vi "main.vi"() -> ()   [LabVIEW 2018]
doc: "This example demonstrates the use of binary morphological reconstruction in the particle analysis. The example allows you to keep the particles completely inside the ROI, completely outside the ROI or on the ROI."
uses:
  <vilib>/vision/NI_Vision_Development_Module.lvlib
panel:
  out "反射图":T1(plugin-control)
  in  "Font, Size & Style 3":T2={"Desired Font (Application)"=enum."Application Font", "[User-specified Font]"={"Font Name"="", "Size"=12, "Strikeout?"=FALSE, "Italic?"=FALSE, "Underline?"=FALSE, "Outline?"=FALSE, "Shadow?"=FALSE, "Bold?"=FALSE, "Rotation Angle"=0.0}, "Horizontal Alignment"=0, "Vertical Alignment"=0} {"Vertical Alignment" items=["Bottom", "Top", "Baseline"]; "Horizontal Alignment" items=["Left", "Center", "Right"]; "[User-specified Font]"."Rotation Angle" format="%.2f"}
  out "最大灰度值":sgl
  out "全图灰度级信息":T3 {"标准差" format="%.2f"; "均值" format="%.2f"; "相邻灰度级间隔" format="%.2f"; "起始灰度值" format="%.2f"; "最大值" format="%.2f"; "最小值" format="%.2f"}
  out "最大灰度值":sgl
  out "反射图灰度表":u32[](graph)
  in  "预处理":bool
  in  "查看标注":bool
  in  "导入图像":bool
  in  "删除标注":bool
  in  "退出":bool
  out "标注框总数":dbl
  out "全图灰度级信息":T3 {"标准差" format="%.2f"; "均值" format="%.2f"; "相邻灰度级间隔" format="%.2f"; "起始灰度值" format="%.2f"; "最大值" format="%.2f"; "最小值" format="%.2f"}
  out "穿透图灰度表":u32[](graph)
  in  "Font, Size & Style 2":T2={"Desired Font (Application)"=enum."Application Font", "[User-specified Font]"={"Font Name"="", "Size"=12, "Strikeout?"=FALSE, "Italic?"=FALSE, "Underline?"=FALSE, "Outline?"=FALSE, "Shadow?"=FALSE, "Bold?"=FALSE, "Rotation Angle"=0.0}, "Horizontal Alignment"=0, "Vertical Alignment"=0} {"Vertical Alignment" items=["Bottom", "Top", "Baseline"]; "Horizontal Alignment" items=["Left", "Center", "Right"]; "[User-specified Font]"."Rotation Angle" format="%.2f"}
  in  "Font, Size & Style":T2={"Desired Font (Application)"=enum."Application Font", "[User-specified Font]"={"Font Name"="", "Size"=12, "Strikeout?"=FALSE, "Italic?"=FALSE, "Underline?"=FALSE, "Outline?"=FALSE, "Shadow?"=FALSE, "Bold?"=FALSE, "Rotation Angle"=0.0}, "Horizontal Alignment"=0, "Vertical Alignment"=0} {"Vertical Alignment" items=["Bottom", "Top", "Baseline"]; "Horizontal Alignment" items=["Left", "Center", "Right"]; "[User-specified Font]"."Rotation Angle" format="%.2f"}
  out "框组":T4(array[cluster])
  in  "Operation":enum16{"overlay rectangle"}(ring)
  out "标注图":T1(plugin-control)
  # "穿透法图像"
  # "反射法图像"
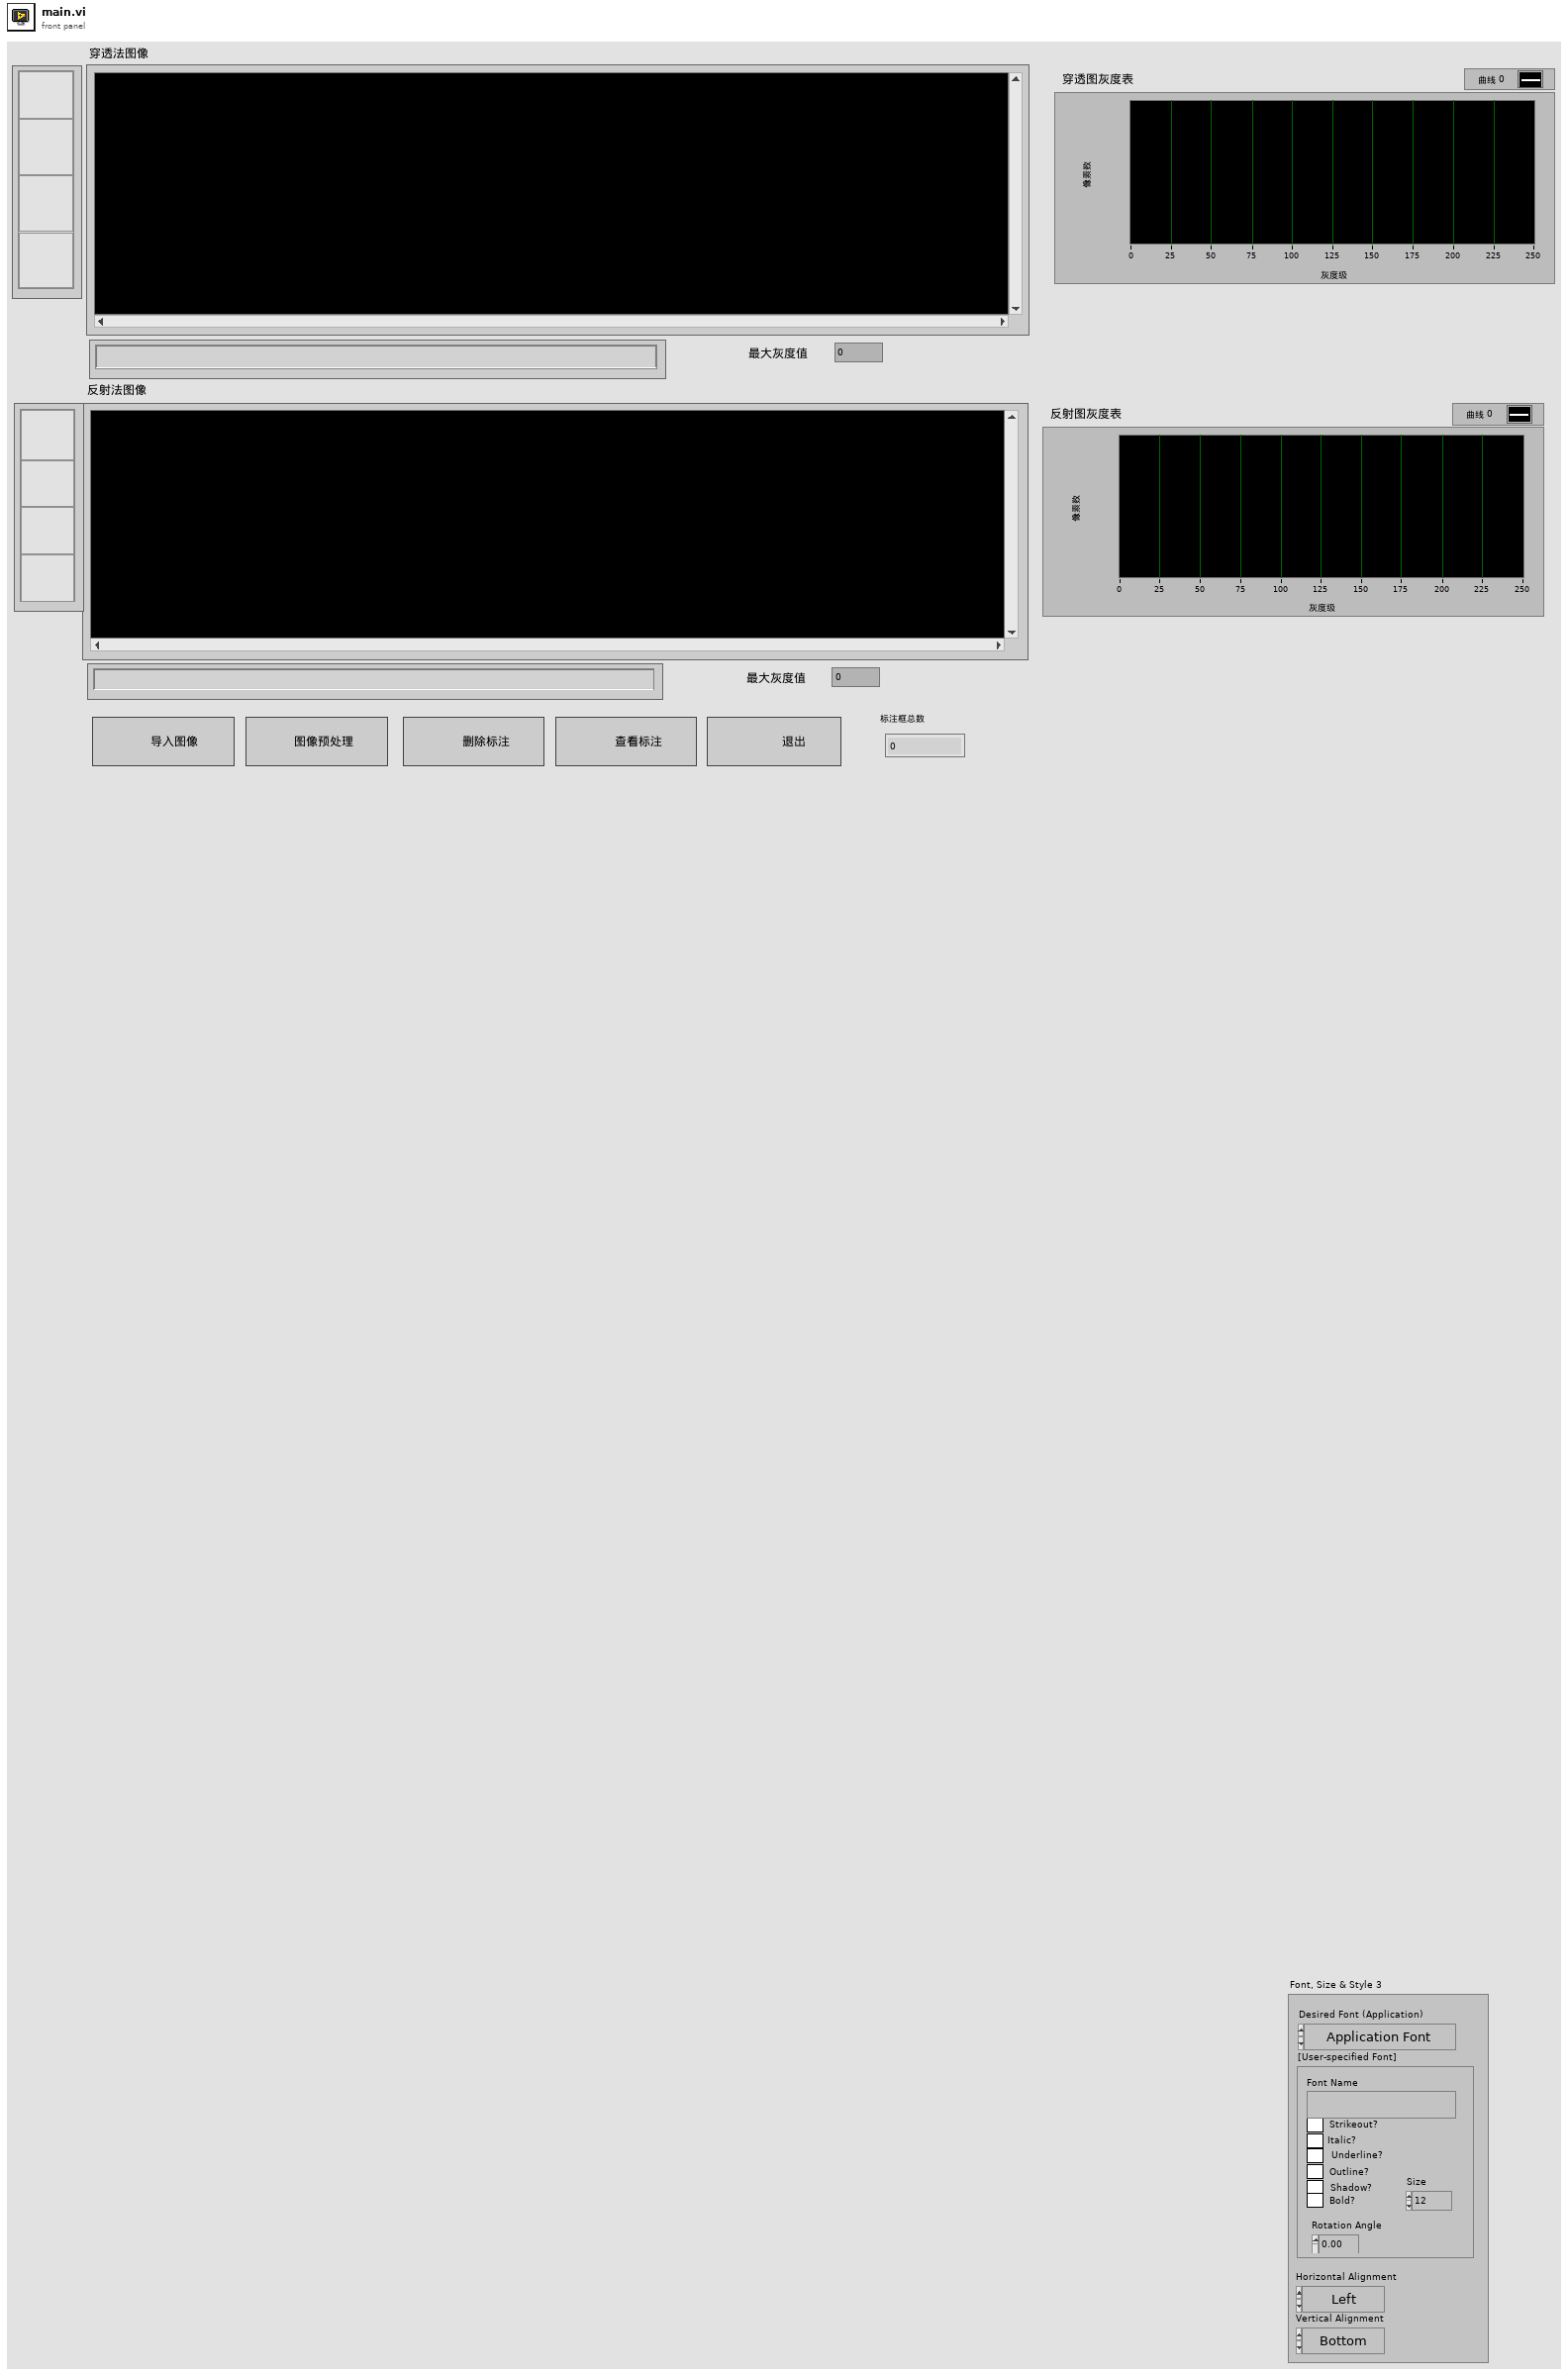
[diagram p1: front panel]
types:
  T1 = typedef "IMAQ Image.ctl" = refnum<image>
  T2 = cluster{"Desired Font (Application)":enum16{"User-specified Font", "Application Font", "System Font", "Dialog Font"}, "[User-specified Font]":cluster{"Font Name":string, "Size":i16, "Strikeout?":bool, "Italic?":bool, "Underline?":bool, "Outline?":bool, "Shadow?":bool, "Bold?":bool, "Rotation Angle":dbl}, "Horizontal Alignment":i16, "Vertical Alignment":i16}
  T3 = cluster{"histogram":u32[], "最小值":sgl, "最大值":sgl, "起始灰度值":sgl, "相邻灰度级间隔":sgl, "均值":sgl, "标准差":sgl, "像素面积":i32}
  T4 = cluster{"Global Rectangle":i32[], "Contours":cluster{"Contour Type":u32, "ROI Type":u32, "Points":i32[]}[]}[]
  T5 = typedef "Image Type" = u32
  T6 = cluster{"Global Rectangle":i32[], "Contours":cluster{"Contour Type":u32, "ROI Type":u32, "Points":i32[]}[]}
  T7 = cluster{"histogram":u32[], "Minimal Value":sgl, "Maximal Value":sgl, "Starting Value":sgl, "Interval Width":sgl, "Mean Value":sgl, "Standard  Variation":sgl, "Area (pixels)":i32}
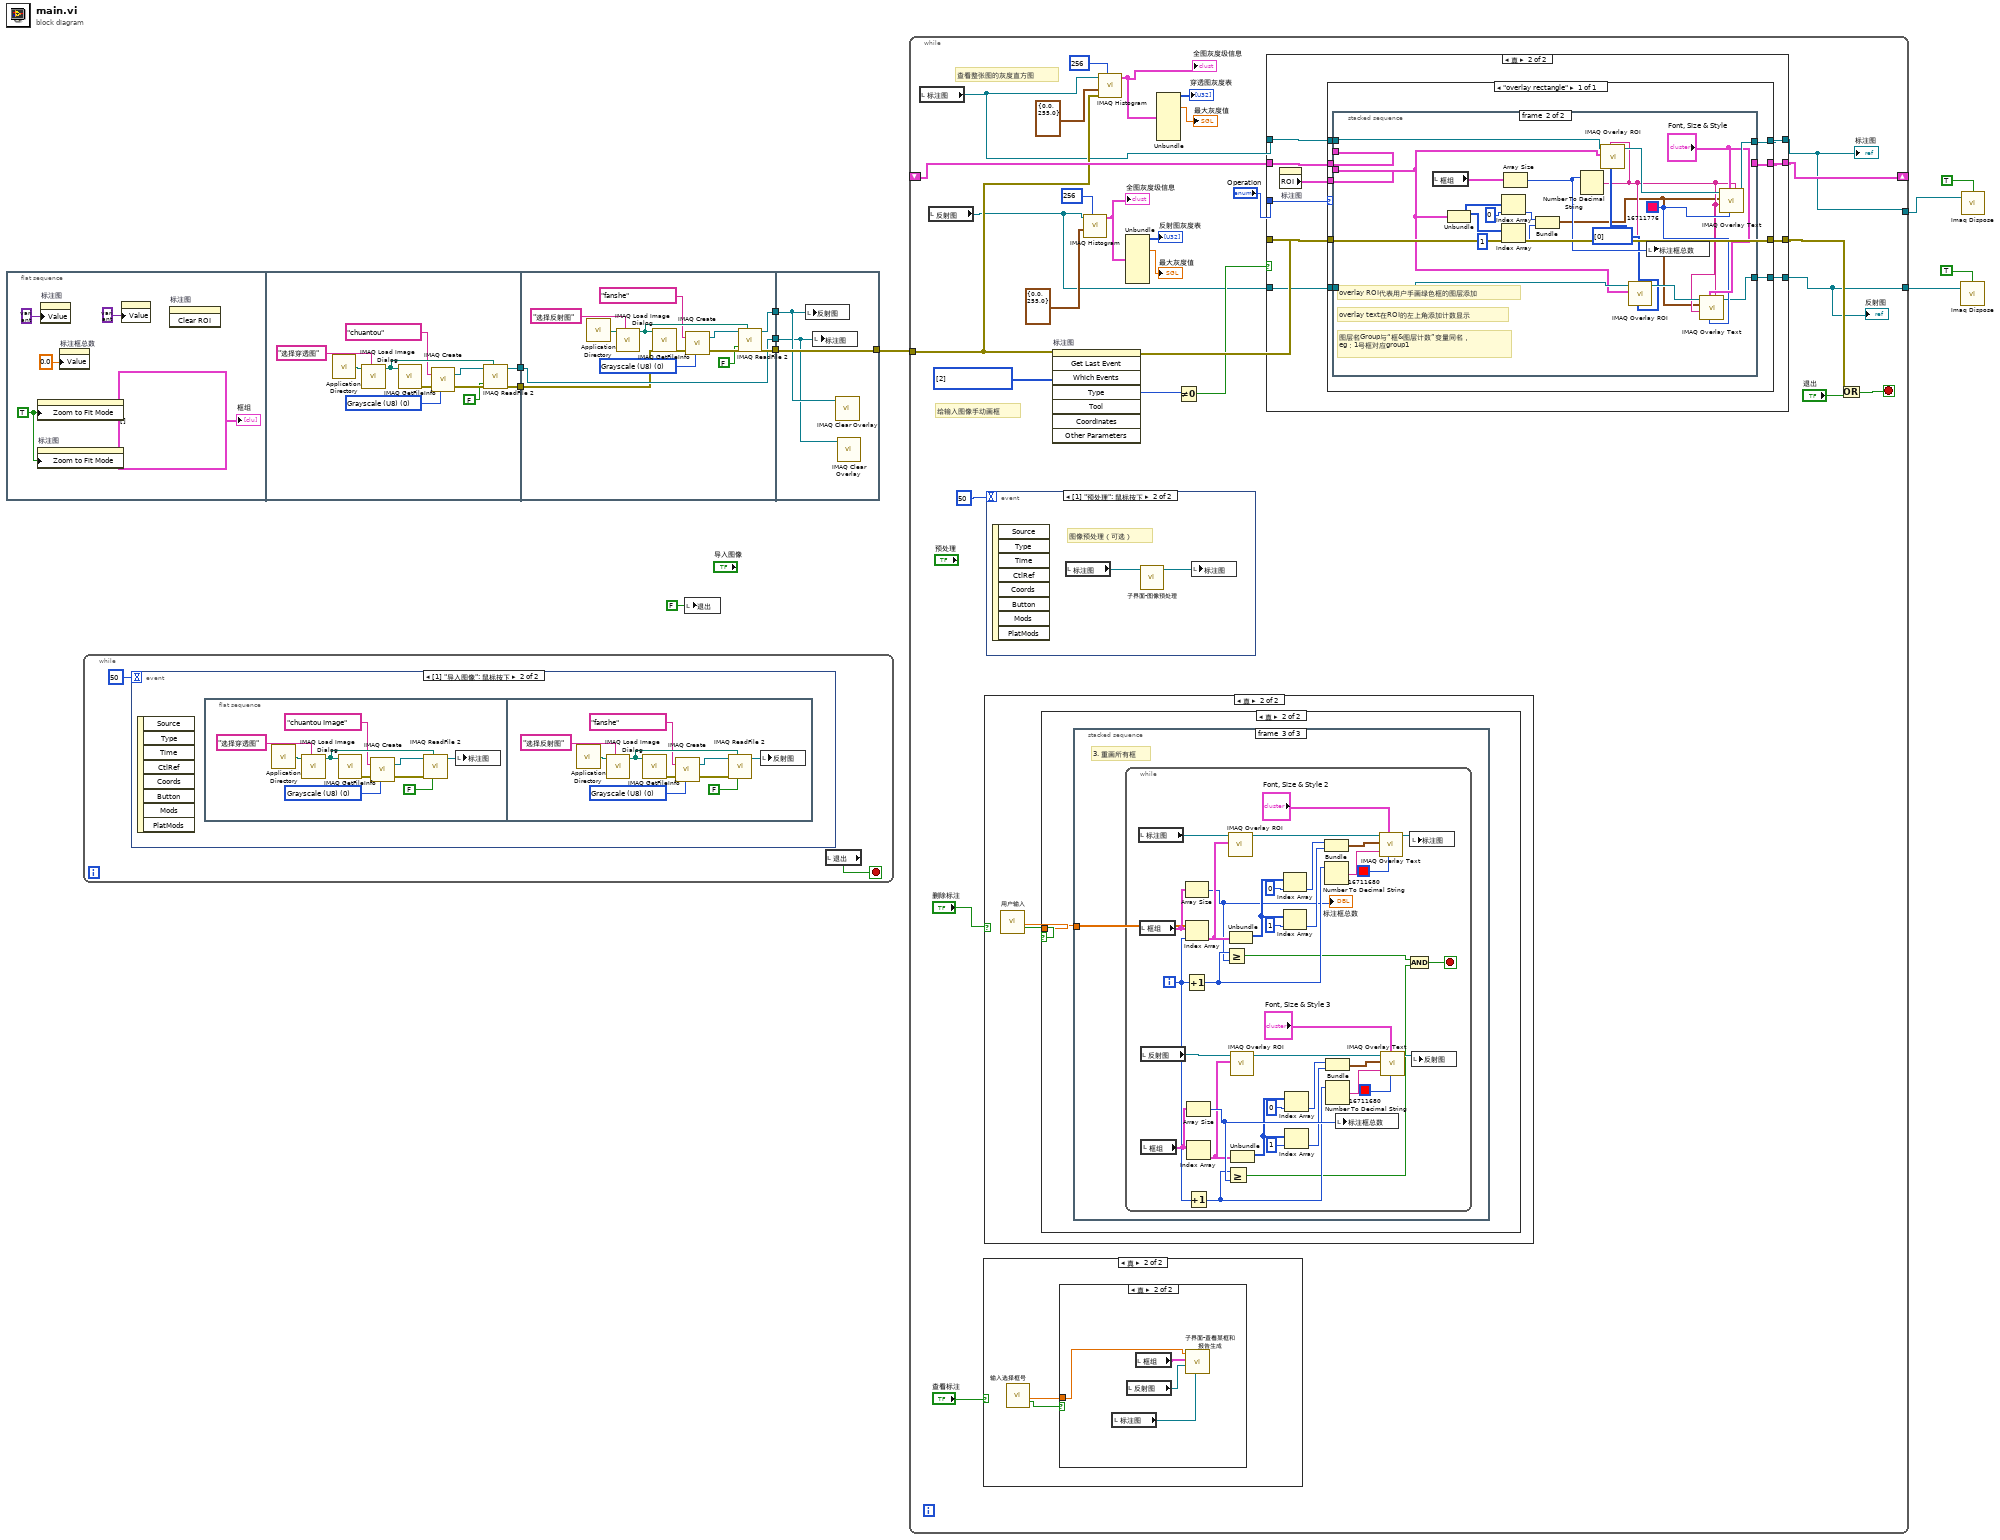
[diagram p0: block diagram]
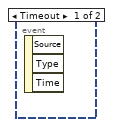
[diagram p2: hidden frame]
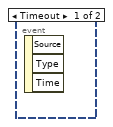
[diagram p3: hidden frame]
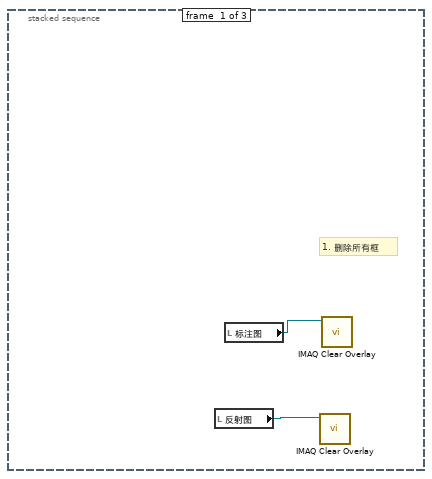
[diagram p8: hidden frame]
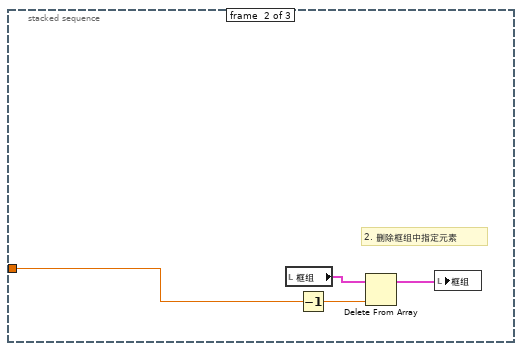
[diagram p9: hidden frame]
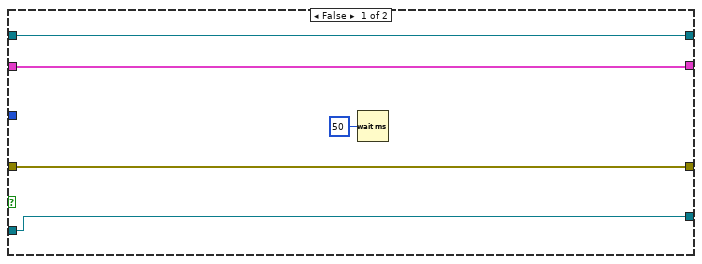
[diagram p10: hidden frame]
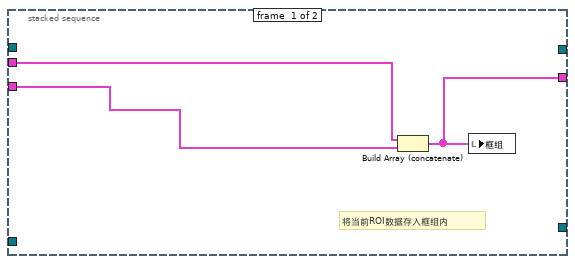
[diagram p11: hidden frame]
diagram:
  n1 = flat-sequence {
    tunnel: [w18] -> w8
    tunnel: [w17] -> w7
    tunnel: w8 -> [w29]
    tunnel: w7 -> [w30]
    tunnel: [w31] -> w6
    tunnel: [w30] -> w5
    tunnel: [w28] -> w4
    tunnel: [w43] -> w11
    tunnel: w6 -> [w43]
    tunnel: w5 -> [w41]
    tunnel: w4 -> [w42]
    frame #0 {
      w15 = TRUE ("Zoom to Fit Mode")
      n2 = property on="反射图" class="ImageControl"("Zoom to Fit Mode"=w15) -> ()  [unwired: 2 in, 2 out]
      n3 = property on="标注图" class="ImageControl"("Zoom to Fit Mode"=w15) -> ()  [unwired: 2 in, 2 out]
      n4 = property on="标注图" class="ImageControl"("Value"=variant ("值")) -> ()  [unwired: 2 in, 2 out]
      n5 = property on="标注框总数" class="DigNum (严格)"("Value"=0.0 ("标注框总数")) -> ()  [unwired: 2 in, 2 out]
      n6 = property on="反射图" class="ImageControl"("Value"=variant ("值")) -> ()  [unwired: 2 in, 2 out]
      n7 = invoke on="标注图" class="ImageControl" method="Clear ROI"() -> ()  [unwired: 3 in, 3 out]
      "框组" <- T4 [] ("框组")
    }
    frame #1 {
      w19 = T5 0 items=["Grayscale (U8)", "Grayscale (I16)", "Grayscale (SGL)", "Complex (CSG)", "RGB (U32)", "HSL (U32)", "RGB (U64)", "Grayscale (U16)"] ("Image Type")
      n8 = call <vilib>:"Application Directory.vi"() -> ("Application Directory"=w27:path)
      n9 = call "IMAQ Load Image Dialog"("Prompt"="选择穿透图" ("prompt"), "Start Path"=w27) -> ("Path"=w23:path)  [unwired: 7 in, 2 out]
      n10 = call "IMAQ GetFileInfo"("File Path"=w23) -> ("error out"=w24:errorcluster)  [unwired: 4 in, 6 out]
      n11 = call "IMAQ Create"("Image Name"="chuantou", "Image Type"=w19, "error in (no error)"=w24) -> ("New Image"=w25:T1, "error out"=w26:errorcluster)  [unwired: 2 in]
      n12 = call "IMAQ ReadFile 2"("Use File Path Image Type"=FALSE, "File Path"=w23, "error in (no error)"=w26, "Image"=w25) -> ("error out"=w18:errorcluster, "Image Out"=w17:T1)  [unwired: 3 in, 3 out]
    }
    frame #2 {
      w32 = T5 0 items=["Grayscale (U8)", "Grayscale (I16)", "Grayscale (SGL)", "Complex (CSG)", "RGB (U32)", "HSL (U32)", "RGB (U64)", "Grayscale (U16)"] ("Image Type")
      n13 = call <vilib>:"Application Directory.vi"() -> ("Application Directory"=w40:path)
      n14 = call "IMAQ Load Image Dialog"("Prompt"="选择反射图" ("prompt"), "Start Path"=w40) -> ("Path"=w36:path)  [unwired: 7 in, 2 out]
      n15 = call "IMAQ GetFileInfo"("error in (no error)"=w29, "File Path"=w36) -> ("error out"=w37:errorcluster)  [unwired: 3 in, 6 out]
      n16 = call "IMAQ Create"("Image Name"="fanshe", "Image Type"=w32, "error in (no error)"=w37) -> ("New Image"=w38:T1, "error out"=w39:errorcluster)  [unwired: 2 in]
      n17 = call "IMAQ ReadFile 2"("Use File Path Image Type"=FALSE, "File Path"=w36, "error in (no error)"=w39, "Image"=w38) -> ("error out"=w31:errorcluster, "Image Out"=w28:T1)  [unwired: 3 in, 3 out]
    }
    frame #3 {
      n18 = local write "反射图"(w42) -> ()
      n19 = local write "标注图"(w41) -> ()
      n20 = call "IMAQ Clear Overlay"("Image"=w42) -> ()  [unwired: 9 in, 2 out]
      n21 = call "IMAQ Clear Overlay"("Image"=w41) -> ()  [unwired: 9 in, 2 out]
    }
  }
  n22 = while {
    stop <- w44 stop-if-true
    n23 = event shown="[1] \"导入图像\": 鼠标按下" {
      selector: _ -> [_ _]
      dyn-events: _ -> [_ _]
      timeout: 50 -> [_ _]
      event Timeout {
        n24 = event-data() -> ()  [unwired: 1 in, 3 out]
      }
      event "导入图像": Mouse Down {
        n25 = event-data() -> ()  [unwired: 1 in, 8 out]
        n26 = flat-sequence {
          frame #0 {
            w47 = T5 0 items=["Grayscale (U8)", "Grayscale (I16)", "Grayscale (SGL)", "Complex (CSG)", "RGB (U32)", "HSL (U32)", "RGB (U64)", "Grayscale (U16)"] ("Image Type")
            n27 = call <vilib>:"Application Directory.vi"() -> ("Application Directory"=w55:path)
            n28 = call "IMAQ Load Image Dialog"("Prompt"="选择穿透图" ("prompt"), "Start Path"=w55) -> ("Path"=w51:path)  [unwired: 7 in, 2 out]
            n29 = call "IMAQ GetFileInfo"("File Path"=w51) -> ("error out"=w52:errorcluster)  [unwired: 4 in, 6 out]
            n30 = call "IMAQ Create"("Image Name"="chuantou Image", "Image Type"=w47, "error in (no error)"=w52) -> ("New Image"=w53:T1, "error out"=w54:errorcluster)  [unwired: 2 in]
            n31 = call "IMAQ ReadFile 2"("Use File Path Image Type"=FALSE, "File Path"=w51, "error in (no error)"=w54, "Image"=w53) -> ("Image Out"=w46:T1)  [unwired: 3 in, 4 out]
            n32 = local write "标注图"(w46) -> ()
          }
          frame #1 {
            w59 = T5 0 items=["Grayscale (U8)", "Grayscale (I16)", "Grayscale (SGL)", "Complex (CSG)", "RGB (U32)", "HSL (U32)", "RGB (U64)", "Grayscale (U16)"] ("Image Type")
            n33 = call <vilib>:"Application Directory.vi"() -> ("Application Directory"=w61:path)
            n34 = call "IMAQ Load Image Dialog"("Prompt"="选择反射图" ("prompt"), "Start Path"=w61) -> ("Path"=w65:path)  [unwired: 7 in, 2 out]
            n35 = call "IMAQ GetFileInfo"("File Path"=w65) -> ("error out"=w64:errorcluster)  [unwired: 4 in, 6 out]
            n36 = call "IMAQ Create"("Image Name"="fanshe", "Image Type"=w59, "error in (no error)"=w64) -> ("New Image"=w63:T1, "error out"=w62:errorcluster)  [unwired: 2 in]
            n37 = call "IMAQ ReadFile 2"("Use File Path Image Type"=FALSE, "File Path"=w65, "error in (no error)"=w62, "Image"=w63) -> ("Image Out"=w56:T1)  [unwired: 3 in, 4 out]
            n38 = local write "反射图"(w56) -> ()
          }
        }
      }
    }
    n39 = local read "退出"() -> (w44:bool)
  }
  n40 = local write "退出"(FALSE ("退出")) -> ()
  n41 = while {
    shift-right: [w86] -> _
    shift-left: _ -> [w85]
    tunnel: w11 -> [w84]
    tunnel: [w66] -> w9
    tunnel: [w67] -> w2
    stop <- w88 stop-if-true
    w91 = i32[] [2] items=["No Event"=0, "Click Event"=1, "Draw Event"=2, "Size Event"=4, "Scroll Event"=5, "Double Click Event"=8] ("Which Events")
    # "给输入图像手动画框"
    # "查看整张图的灰度直方图"
    n42 = local read "标注图"() -> (w68:T1)
    n43 = local read "反射图"() -> (w69:T1)
    n44 = case shown="真" "查看标注" {
      frame False {
      }
      frame True {
        n45 = call "输入选择框号"() -> ("框号"=w97:dbl, "确定"=w96:bool)  [unwired: 17 in, 1 out]
        n46 = case shown="真" w96 {
          tunnel: w97 -> [_ w101]
          frame False {
            # "用户取消操作"
          }
          frame True {
            n47 = local read "标注图"() -> (w98:T1)
            n48 = local read "反射图"() -> (w99:T1)
            n49 = local read "框组"() -> (w100:T4)
            n50 = call "子界面-查看某框和报告生成.vi"("框号"=w101, "框组"=w100, "反射图"=w99, "标注图"=w98) -> ()  [unwired: 2 in]
          }
        }
      }
    }
    n51 = case shown="真" "删除标注" {
      frame False {
      }
      frame True {
        n52 = call "用户输入"() -> ("框号"=w102:dbl, "确定"=w103:bool)  [unwired: 17 in, 1 out]
        n53 = case shown="真" w103 {
          tunnel: w102 -> [_ w104]
          frame False {
            # "用户取消操作"
          }
          frame True {
            n54 = stacked-sequence {
              tunnel: w104 -> [_ w109 _]
              frame #0 {
                # "1. 删除所有框"
                n55 = local read "反射图"() -> (w105:T1)
                n56 = local read "标注图"() -> (w106:T1)
                n57 = call "IMAQ Clear Overlay"("Image"=w105) -> ()  [unwired: 9 in, 2 out]
                n58 = call "IMAQ Clear Overlay"("Image"=w106) -> ()  [unwired: 9 in, 2 out]
              }
              frame #1 {
                # "2. 删除框组中指定元素"
                n59 = local read "框组"() -> (w110:T4)
                n60 = Decrement(x=w109) -> (x-1=w108:dbl)
                n61 = Delete From Array(array=w110, index=w108) -> (array with subset deleted=w107:T4)  [unwired: 1 in, 1 out]
                n62 = local write "框组"(w107) -> ()
              }
              frame #2 {
                # "3. 重画所有框"
                n63 = while {
                  i -> [w114]
                  stop <- w111 stop-if-true
                  n64 = local read "标注图"() -> (w146:T1)
                  n65 = local read "框组"() -> (w140:T4)
                  n66 = local read "反射图"() -> (w115:T1)
                  n67 = local read "框组"() -> (w121:T4)
                  n68 = Array Size(array=w140) -> (size(s)=w131:i32)
                  "标注框总数" <- w131
                  n69 = Index Array(array=w140, index=w114) -> (element=w133:T6)
                  n70 = Increment(x=w114) -> (x+1=w145:i32)
                  n71 = Array Size(array=w121) -> (size(s)=w130:i32)
                  n72 = Index Array(array=w121) -> (element=w128:T6)  [unwired: 1 in]
                  n73 = Increment(x=w114) -> (x+1=w116:i32)
                  n74 = Greater Or Equal?(x=w145, y=w131) -> (x >= y?=w113:bool)
                  n75 = Greater Or Equal?(x=w116, y=w130) -> (x >= y?=w112:bool)
                  n76 = call "IMAQ Overlay ROI"("ROI Descriptor"=w133, "Image"=w146) -> ("Image Out"=w142:T1)  [unwired: 8 in, 1 out]
                  n77 = Unbundle(w133) -> ("Global Rectangle"=w136:i32[])  [unwired: 1 out]
                  n78 = call "IMAQ Overlay ROI"("ROI Descriptor"=w128, "Image"=w115) -> ("Image Out"=w119:T1)  [unwired: 8 in, 1 out]
                  n79 = Unbundle(w128) -> ("Global Rectangle"=w125:i32[])  [unwired: 1 out]
                  n80 = Index Array(array=w136, index=0 ("索引")) -> (element=w137:i32)
                  n81 = Index Array(array=w136, index=1 ("索引")) -> (element=w138:i32)
                  n82 = Index Array(array=w125, index=0 ("索引")) -> (element=w124:i32)
                  n83 = Index Array(array=w125, index=1 ("索引")) -> (element=w123:i32)
                  n84 = Bundle(w137, w138) -> (w135:cluster{i32, i32})  [unwired: 1 in]
                  n85 = Number To Decimal String(number=w145) -> (decimal integer string=w143:string)  [unwired: 1 in]
                  n86 = Bundle(w124, w123) -> (w126:cluster{i32, i32})  [unwired: 1 in]
                  n87 = Number To Decimal String(number=w116) -> (decimal integer string=w118:string)  [unwired: 1 in]
                  n88 = local write "标注框总数"(w130) -> ()
                  n89 = call "IMAQ Overlay Text"("Text Color (black)"=u32 16711680, "Font, Size & Style"="Font, Size & Style 2", "String"=w143, "Origin"=w135, "Image"=w142) -> ("Image Out"=w141:T1)  [unwired: 5 in, 1 out]
                  n90 = call "IMAQ Overlay Text"("Text Color (black)"=u32 16711680, "Font, Size & Style"="Font, Size & Style 3", "String"=w118, "Origin"=w126, "Image"=w119) -> ("Image Out"=w120:T1)  [unwired: 5 in, 1 out]
                  n91 = And(x=w113, y=w112) -> (x .and. y?=w111:bool)
                  n92 = local write "标注图"(w141) -> ()
                  n93 = local write "反射图"(w120) -> ()
                }
              }
            }
          }
        }
      }
    }
    n94 = event shown="[1] \"预处理\": 鼠标按下" {
      selector: _ -> [_ _]
      dyn-events: _ -> [_ _]
      timeout: 50 -> [_ _]
      event Timeout {
        n95 = event-data() -> ()  [unwired: 1 in, 3 out]
      }
      event "预处理": Mouse Down {
        # "图像预处理（可选）"
        n96 = event-data() -> ()  [unwired: 1 in, 8 out]
        n97 = local read "标注图"() -> (w95:T1)
        n98 = call "子界面-图像预处理.vi"("原图"=w95) -> ("处理后"=w94:T1)  [unwired: 10 in]
        n99 = local write "标注图"(w94) -> ()
      }
    }
    n100 = invoke on="标注图" class="ImageControl" method="Get Last Event"(error in=w84, "Which Events"=w91) -> (error out=w90:errorcluster, "Type"=w92:i32)  [unwired: 6 in, 6 out]
    n101 = call "IMAQ Histogram"("Number of Classes"=256, "Interval Range"=cluster{"Minimum":sgl, "Maximum":sgl} {"Minimum"=0.0, "Maximum"=255.0}, "Image"=w69) -> ("Histogram Report"=w72:T7)  [unwired: 7 in, 1 out]
    "全图灰度级信息" <- w72
    n102 = call "IMAQ Histogram"("Number of Classes"=256, "error in (no error)"=w84, "Interval Range"=cluster{"Minimum":sgl, "Maximum":sgl} {"Minimum"=0.0, "Maximum"=255.0}, "Image"=w68) -> ("Histogram Report"=w75:T7)  [unwired: 6 in, 1 out]
    "全图灰度级信息" <- w75
    n103 = Unbundle(w72) -> ("histogram"=→"反射图灰度表":u32[], "Maximal Value"=→"最大灰度值":sgl)  [unwired: 6 out]
    n104 = Unbundle(w75) -> ("histogram"=→"穿透图灰度表":u32[], "Maximal Value"=→"最大灰度值":sgl)  [unwired: 6 out]
    n105 = Not Equal To 0?(x=w92) -> (x != 0?=w87:bool)
    n106 = case shown="真" w87 {
      tunnel: w68 -> [w151 w161]
      tunnel: [w151 w160] -> w66
      tunnel: "Operation" -> [_ w158]
      tunnel: w90 -> [w150 w157]
      tunnel: [w150 w156] -> w89
      tunnel: [w148 w155] -> w86
      tunnel: w85 -> [w148 w154]
      tunnel: w69 -> [w147 w153]
      tunnel: [w147 w152] -> w67
      frame False {
        n107 = Wait (ms)(milliseconds to wait=u32 50) -> ()  [unwired: 1 out]
      }
      frame True {
        n108 = property on="标注图" class="ImageControl"() -> ("ROI"=w159:T6)  [unwired: 2 in, 2 out]
        n109 = case shown="\"overlay rectangle\"" w158 {
          tunnel: w161 -> [w168]
          tunnel: w159 -> [w166]
          tunnel: [w167] -> w160
          tunnel: w157 -> [w169]
          tunnel: [w169] -> w156
          tunnel: [w165] -> w155
          tunnel: w154 -> [w164]
          tunnel: w153 -> [w163]
          tunnel: [w162] -> w152
          frame "overlay rectangle" {
            n110 = stacked-sequence {
              tunnel: w168 -> [_ w184]
              tunnel: [_ w183] -> w167
              tunnel: w166 -> [w172 w180]
              tunnel: [w170 _] -> w165
              tunnel: w164 -> [w171 _]
              tunnel: w163 -> [_ w181]
              tunnel: [_ w177] -> w162
              frame #0 {
                # "将当前ROI数据存入框组内"
                n111 = Build Array (concatenate)(w171, w172) -> (w170:T4)
                n112 = local write "框组"(w170) -> ()
              }
              frame #1 {
                w175 = u32[] [0] ("Colors (Green)")
                w178 = u32 16711776 ("Text Color (black)")
                # "图层名Group与“框&图层计数”变量同名，\neg：1号框对应group1"
                # "overlay text在ROI的左上角添加计数显示"
                # "overlay ROI代表用户手画绿色框的图层添加"
                n113 = local read "框组"() -> (w187:T4)
                n114 = Unbundle(w180) -> ("Global Rectangle"=w190:i32[])  [unwired: 1 out]
                n115 = Index Array(array=w190, index=0 ("索引")) -> (element=w189:i32)
                n116 = Index Array(array=w190, index=1 ("索引")) -> (element=w188:i32)
                n117 = Array Size(array=w187) -> (size(s)=w182:i32)
                n118 = Bundle(w189, w188) -> (w173:cluster{i32, i32})  [unwired: 1 in]
                n119 = Number To Decimal String(number=w182) -> (decimal integer string=w174:string)  [unwired: 1 in]
                n120 = call "IMAQ Overlay ROI"("Colors (Green)"=w175, "Group"=w174, "ROI Descriptor"=w180, "Image"=w184) -> ("Image Out"=w191:T1)  [unwired: 6 in, 1 out]
                n121 = call "IMAQ Overlay ROI"("Colors (Green)"=w175, "Group"=w174, "ROI Descriptor"=w180, "Image"=w181) -> ("Image Out"=w176:T1)  [unwired: 6 in, 1 out]
                n122 = local write "标注框总数"(w182) -> ()
                n123 = call "IMAQ Overlay Text"("Group"=w174, "Text Color (black)"=w178, "Font, Size & Style"="Font, Size & Style", "String"=w174, "Origin"=w173, "Image"=w176) -> ("Image Out"=w177:T1)  [unwired: 4 in, 1 out]
                n124 = call "IMAQ Overlay Text"("Group"=w174, "Text Color (black)"=w178, "Font, Size & Style"="Font, Size & Style", "String"=w174, "Origin"=w173, "Image"=w191) -> ("Image Out"=w183:T1)  [unwired: 4 in, 1 out]
              }
            }
          }
        }
      }
    }
    "标注图" <- w66
    "反射图" <- w67
    n125 = Or(x=w89, y="退出") -> (x .or. y?=w88:bool)
  }
  n126 = call "Imaq Dispose"("All Images? (No)"=TRUE, "Image"=w2) -> ()  [unwired: 1 in, 4 out]
  n127 = call "Imaq Dispose"("All Images? (No)"=TRUE, "Image"=w9) -> ()  [unwired: 1 in, 4 out]
